vi "TestWebService.vi"() -> ()   [LabVIEW 2017]
uses:
  E:/Earcup/Dyson Earcup Flow Program V1.0.0-0202-DLL2.0/SubVIs/WebService/EquipmentWebService.dll
  EquipmentWebService.dll
  EquipmentWebService.lvlib
panel:
  out "TestComplect Out":T1
  in  "TestComplete in":T2={"overllResult"="PASS", "resourceCode"="G571L102", "serialNumber"="C012496", "site"="C012", "specCode"="UKAM1006", "Data"=[]}
  out "testStart Out":T1
  in  "TestStart in":T3={"btAddressReq"=FALSE, "resourceCode"="G571L102", "serialNumber"="C012496", "site"="C012", "specCode"="UKAM1006"}
  in  "Proxy Server Settings":T4={"Address"="192.168.50.95", "Port"=50000, "Username"="", "Password"="", "Domain"=""}
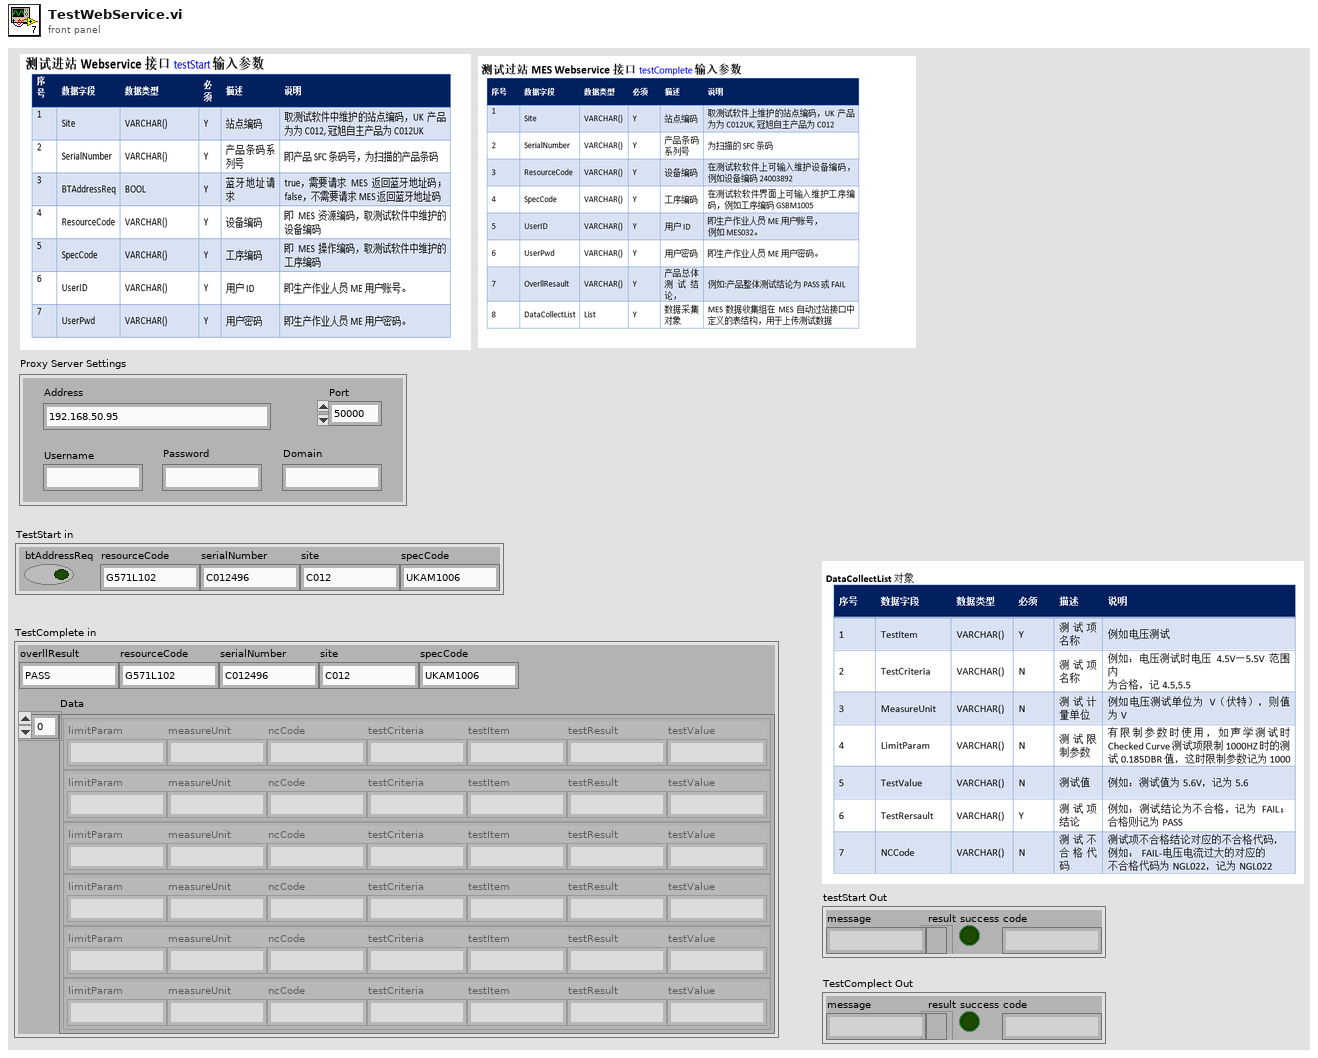
[diagram p1: front panel]
types:
  T1 = cluster{"message":string, "result":refnum<k24>, "success":bool, "code":string}
  T2 = cluster{"overllResult":string, "resourceCode":string, "serialNumber":string, "site":string, "specCode":string, "Data":cluster{"limitParam":string, "measureUnit":string, "ncCode":string, "testCriteria":string, "testItem":string, "testResult":string, "testValue":string}[]}
  T3 = cluster{"btAddressReq":bool, "resourceCode":string, "serialNumber":string, "site":string, "specCode":string}
  T4 = cluster{"Address":string, "Port":u32, "Username":string, "Password":string, "Domain":string}
  T5 = cluster{"limitParam":string, "measureUnit":string, "ncCode":string, "testCriteria":string, "testItem":string, "testResult":string, "testValue":string}[]
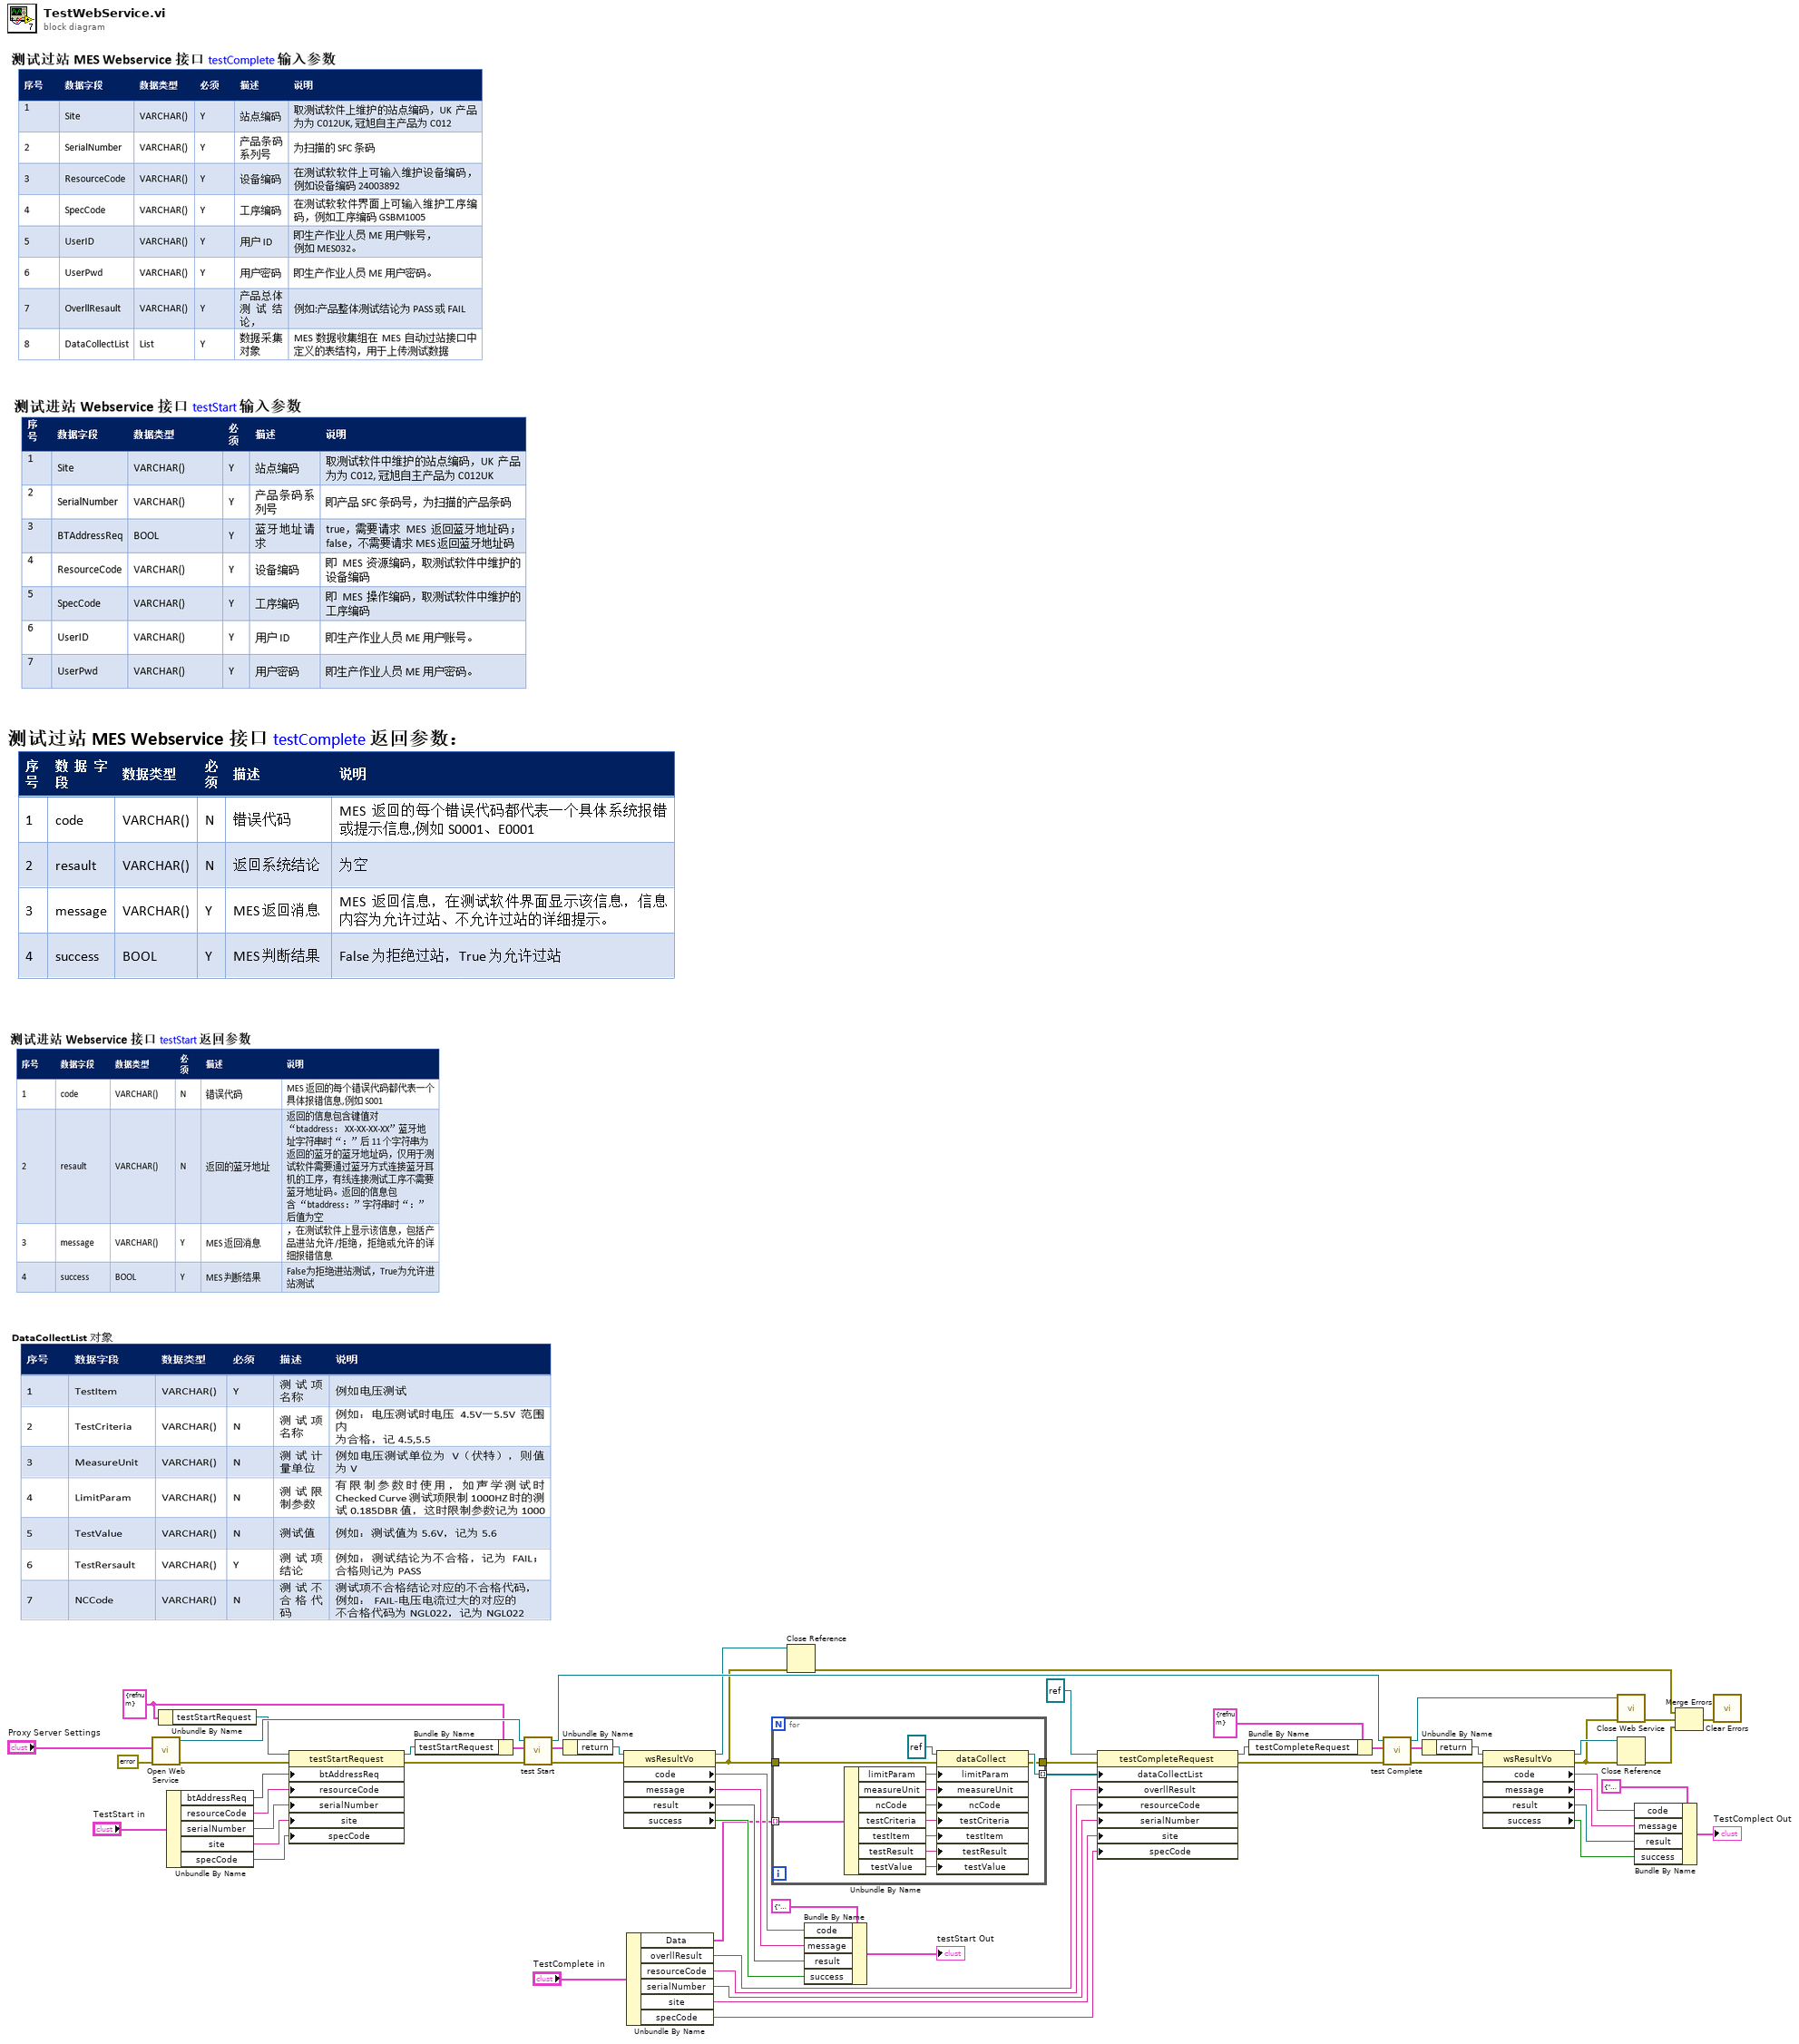
[diagram p0: block diagram]
diagram:
  w5 = cluster{"testStartRequest":refnum<k24>} {"testStartRequest"=refnum} (".NET:EquipmentWebService.testStart")
  n1 = call "Open Web Service.vi"("error in (no error)"=errorcluster {"status"=FALSE, "code"=0, "source"=""}, "Proxy Server Settings"="Proxy Server Settings") -> ("error out"=w7:errorcluster, "EquipmentWebService refnum"=w56:refnum<k24>)  [unwired: 8 in]
  n2 = Unbundle By Name(w5) -> ("testStartRequest"=w1:refnum<k24>)
  n3 = Unbundle By Name("TestStart in") -> ("btAddressReq"=w50:bool, "resourceCode"=w49:string, "serialNumber"=w48:string, "site"=w47:string, "specCode"=w46:string)
  n4 = property class="testStartRequest"(reference=w1, error in=w7, "btAddressReq"=w50, "resourceCode"=w49, "serialNumber"=w48, "site"=w47, "specCode"=w46) -> (reference out=w54:refnum<k24>, error out=w4:errorcluster)
  n5 = Bundle By Name(cluster=w5, "testStartRequest"=w54) -> (w55:cluster{"testStartRequest":refnum<k24>})
  n6 = call "test Start.vi"("error in (no error)"=w4, ".NET:EquipmentWebService.testStart"=w55, "EquipmentWebService refnum"=w56) -> ("error out"=w18:errorcluster, ".NET:EquipmentWebService.testStartResponse"=w53:cluster{"return":refnum<k24>}, "EquipmentWebService refnum out"=w39:refnum<k24>)  [unwired: 6 in]
  n7 = Unbundle By Name(w53) -> ("return"=w52:refnum<k24>)
  n8 = property class="wsResultVo"(reference=w52, error in=w18) -> (reference out=w15:refnum<k24>, error out=w2:errorcluster, "code"=w43:string, "message"=w42:string, "result"=w41:refnum<k24>, "success"=w40:bool)
  n9 = Unbundle By Name("TestComplete in") -> ("Data"=w9:T5, "overllResult"=w32:string, "resourceCode"=w31:string, "serialNumber"=w30:string, "site"=w29:string, "specCode"=w28:string)
  n10 = for {
    tunnel: w9 -> [w61] mode=indexing
    tunnel: [w60] -> w8 mode=indexing
    tunnel: w2 -> [w59]
    tunnel: [w58] -> w6
    n11 = Unbundle By Name(w61) -> ("limitParam"=w68:string, "measureUnit"=w67:string, "ncCode"=w66:string, "testCriteria"=w65:string, "testItem"=w64:string, "testResult"=w63:string, "testValue"=w62:string)
    n12 = property class="dataCollect"(reference=refnum<k24> refnum, error in=w59, "limitParam"=w68, "measureUnit"=w67, "ncCode"=w66, "testCriteria"=w65, "testItem"=w64, "testResult"=w63, "testValue"=w62) -> (reference out=w60:refnum<k24>, error out=w58:errorcluster)
  }
  n13 = Close Reference(reference=w15, error in (no error)=w2) -> (error out=w11:errorcluster)
  n14 = Bundle By Name(cluster=T1 {"message"="", "result"=refnum, "success"=FALSE, "code"=""} ("testStart Out"), "code"=w43, "message"=w42, "result"=w41, "success"=w40) -> (→"testStart Out":T1)
  n15 = property class="testCompleteRequest"(reference=refnum<k24> refnum ("testCompleteRequest"), error in=w6, "dataCollectList"=w8, "overllResult"=w32, "resourceCode"=w31, "serialNumber"=w30, "site"=w29, "specCode"=w28) -> (reference out=w36:refnum<k24>, error out=w3:errorcluster)
  n16 = Bundle By Name(cluster=cluster{"testCompleteRequest":refnum<k24>} {"testCompleteRequest"=refnum} (".NET:EquipmentWebService.testComplete"), "testCompleteRequest"=w36) -> (w35:cluster{"testCompleteRequest":refnum<k24>})
  n17 = call "test Complete.vi"("error in (no error)"=w3, ".NET:EquipmentWebService.testComplete"=w35, "EquipmentWebService refnum"=w39) -> ("error out"=w17:errorcluster, ".NET:EquipmentWebService.testCompleteResponse"=w26:cluster{"return":refnum<k24>}, "EquipmentWebService refnum out"=w27:refnum<k24>)  [unwired: 6 in]
  n18 = Unbundle By Name(w26) -> ("return"=w25:refnum<k24>)
  n19 = property class="wsResultVo"(reference=w25, error in=w17) -> (reference out=w14:refnum<k24>, error out=w13:errorcluster, "code"=w23:string, "message"=w22:string, "result"=w21:refnum<k24>, "success"=w20:bool)
  n20 = call "Close Web Service.vi"("error in (no error)"=w13, "EquipmentWebService refnum"=w27) -> ("error out"=w16:errorcluster)  [unwired: 9 in]
  n21 = Close Reference(reference=w14, error in (no error)=w13) -> (error out=w10:errorcluster)
  n22 = Bundle By Name(cluster=T1 {"message"="", "result"=refnum, "success"=FALSE, "code"=""} ("testStart Out"), "code"=w23, "message"=w22, "result"=w21, "success"=w20) -> (→"TestComplect Out":T1)
  n23 = Merge Errors(w11, w16, w10) -> (w12:errorcluster)
  n24 = call <vilib>:"Clear Errors.vi"("error in (no error)"=w12) -> ()  [unwired: 5 in, 2 out]
